vi "CMD_Close.vi"(0 "reference in":refnum<class "GUI.lvclass">, 11 "error in (no error)":errorcluster) -> (4 "reference out":refnum<class "GUI.lvclass">, 15 "error out":errorcluster)   [LabVIEW 2019, in "GUI.lvclass"]
uses:
  GUI.lvclass
  GUI.lvclass/GUI.ctl
  WindowsState.ctl
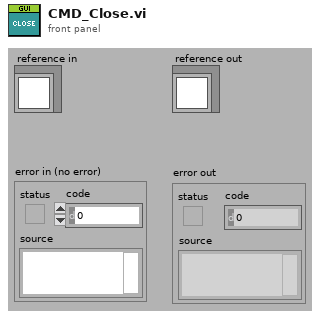
[diagram p1: front panel]
types:
  T1 = typedef "GUI.lvclass/WindowsState.ctl" = enum16{"NotReady", "Ready", "Inserted", "Opened"}
  T2 = typedef "GUI.lvclass/Shered Data.ctl" = cluster{"WindowsState":T1, "UI VI":refnum<vi>, "SubPnl":refnum<vi>}
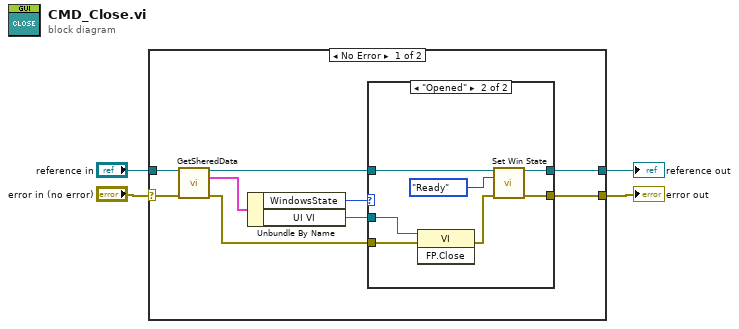
[diagram p0: block diagram]
diagram:
  n1 = case shown="No Error" "error in (no error)" {
    selector: "error in (no error)" -> [w10 w24]
    tunnel: [w13 w24] -> w3
    tunnel: [w12 w23] -> w1
    tunnel: "reference in" -> [w11 w23]
    frame No Error {
      n2 = call "GetSheredData.vi"("reference in"=w11, "error in (no error)"=w10) -> ("reference out"=w8:refnum<class "GUI.lvclass">, "data"=w9:T2, "error out"=w7:errorcluster)  [unwired: 11 in]
      n3 = Unbundle By Name(w9) -> ("WindowsState"=w5:T1, "UI VI"=w6:refnum<vi>)
      n4 = case shown="\"Opened\"" w5 {
        tunnel: w6 -> [_ w22]
        tunnel: w7 -> [w15 w21]
        tunnel: [w15 w19] -> w13
        tunnel: w8 -> [w14 w17]
        tunnel: [w14 w16] -> w12
        frame Default {
        }
        frame "Opened" {
          n5 = invoke class="VI" method="FP.Close"(reference=w22, error in=w21) -> (error out=w20:errorcluster)  [unwired: 1 in, 2 out]
          n6 = call "Set Win State.vi"("reference in"=w17, "WindowsState"=WindowsState."Ready", "error in (no error)"=w20) -> ("reference out"=w16:refnum<class "GUI.lvclass">, "error out"=w19:errorcluster)  [unwired: 11 in]
        }
      }
    }
    frame Error {
    }
  }
  "error out" <- w3
  "reference out" <- w1
